vi "Grid Measurements - Topo & GridSpectr Simple.vi"(6 "Internal use":string, 7 "Grid param":T1 {"height (m)" format="%#_6p"; "width (m)" format="%#_6p"; "center Y (m)" format="%#_6p"; "center X (m)" format="%#_6p"}, 8 "Error in (no error)":errorcluster, 9 "Points Y/Index Y":i32, 10 "Points X/Index X":i32, 11 "Method":enum16{"init", "run", "end"}(ring)) -> (0 "Error out":errorcluster)   [LabVIEW 2014]
doc: "Example of a measurement VI to be used in the \"Experiments on a Grid\" tool as external VI.\n\nThis example measure the topography and spectroscopy data. The spectroscopy measurements are taken on a subgrid. The data are saved to a sxm and a binary file.\n\n- Nanonis Programming Interface -"
uses:
  Instance           1 53Saved   Grid Measurements Example - Topo & GridSpectr .vi
  <userlib>/Nanonis Prog Interface V5/Nanonis Prog Interface.lvlib
panel:
  out "Status":string
  out "Points taken":i32
  in  "Drift correction":i64
  in  "Y subgrid spacing":u16=4
  in  "X subgrid spacing":u16=4
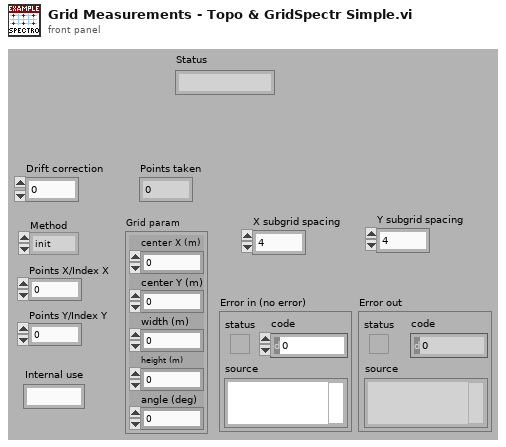
[diagram p1: front panel]
types:
  T1 = cluster{"center X (m)":sgl, "center Y (m)":sgl, "width (m)":sgl, "height (m)":sgl, "angle (deg)":sgl}
  T2 = cluster{"center X":sgl, "center Y":sgl, "angle":sgl, "width":sgl, "height":sgl, "# pixels":i32, "# lines":i32}
  T3 = cluster{"Name":string, "Calibration":sgl, "Offset":sgl, "Channel index":i32}[]
  T4 = cluster{"up/down":bool, "time/line":sgl, "start time":timestamp, "end time":timestamp}
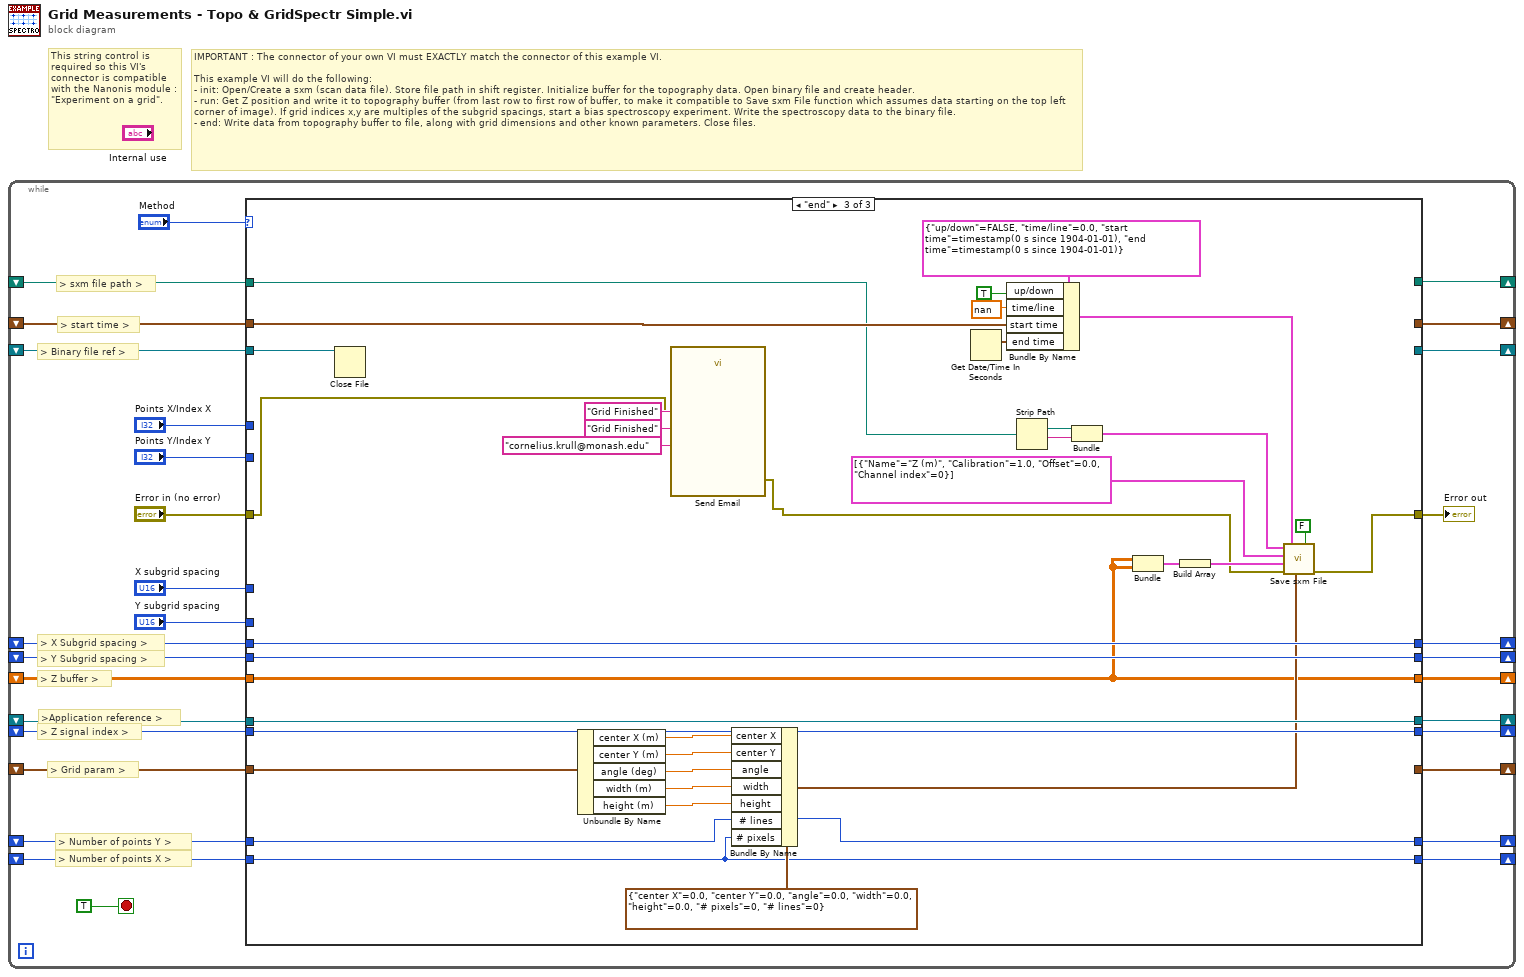
[diagram p0: block diagram]
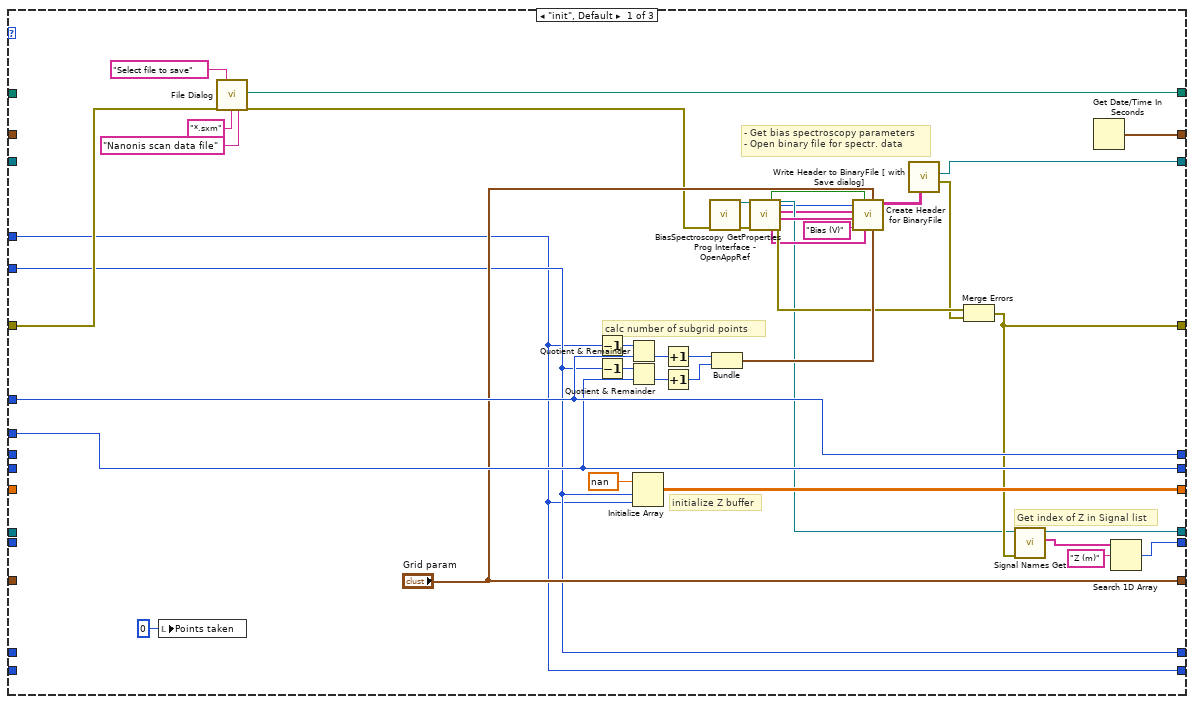
[diagram p2: hidden frame]
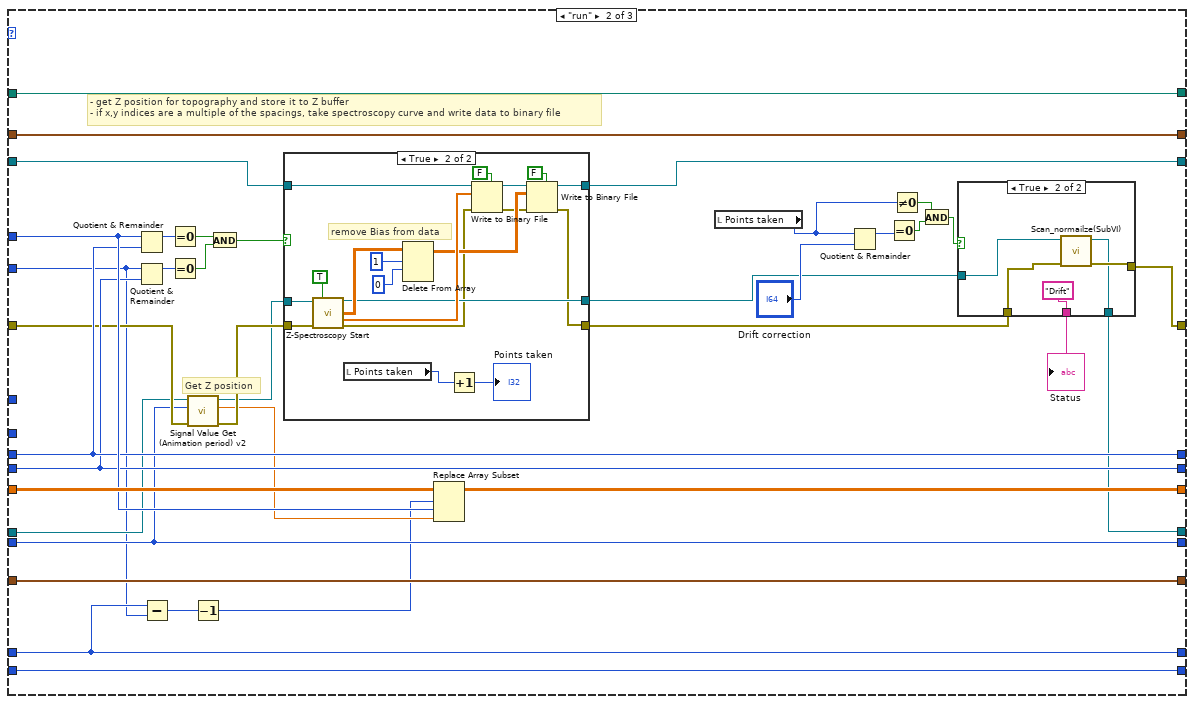
[diagram p3: hidden frame]
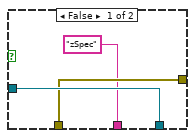
[diagram p4: hidden frame]
diagram:
  # "This string control is required so this VI's connector is compatible with the Nanonis module : \"Experiment on a grid\"."
  # "IMPORTANT : The connector of your own VI must EXACTLY match the connector of this example VI.\n\nThis example VI will do the following:\n- init: Open/Create a sxm (scan data file). Store file path in shift register. Initialize buffer for the topography data. Open binary file and create header.\n- run: Get Z position and write it to topography buffer (from last row to first row of buffer, to make it compatible to Save sxm File function which assumes data starting on the top left corner of image). If grid indices x,y are multiples of the subgrid spacings, start a bias spectroscopy experiment. Write the spectroscopy data to the binary file.\n- end: Write data from topography buffer to file, along with grid dimensions and other known parameters. Close files."
  n1 = while {
    shift-right: [w5] -> _
    shift-left: _ -> [w28]
    shift-right: [w23] -> _
    shift-left: _ -> [w22]
    shift-right: [w20] -> _
    shift-left: _ -> [w21]
    shift-right: [w19] -> _
    shift-left: _ -> [w18]
    shift-right: [w12] -> _
    shift-left: _ -> [w14]
    shift-right: [w13] -> _
    shift-left: _ -> [w15]
    shift-right: [w11] -> _
    shift-left: _ -> [w10]
    shift-right: [w9] -> _
    shift-left: _ -> [w8]
    shift-right: [w7] -> _
    shift-left: _ -> [w6]
    shift-right: [w4] -> _
    shift-left: _ -> [w3]
    shift-right: [w2] -> _
    shift-left: _ -> [w1]
    stop <- TRUE stop-if-true
    # "> Number of points X >"
    # "> Number of points Y >"
    # "> Grid param >"
    # "> start time >"
    # ">Application reference >"
    # "> Y Subgrid spacing >"
    # "> X Subgrid spacing >"
    # "> Z signal index >"
    # "> Binary file ref >"
    # "> Z buffer >"
    # "> sxm file path >"
    n2 = case shown="\"end\"" "Method" {
      tunnel: [w36 w107 _] -> w5
      tunnel: w28 -> [_ w107 w162]
      tunnel: "Error in (no error)" -> [w38 w94 w138]
      tunnel: [w48 w73 w154] -> w26
      tunnel: "Points X/Index X" -> [w32 w102 _]
      tunnel: "Points Y/Index Y" -> [w33 w84 _]
      tunnel: [w70 w105 w143] -> w23
      tunnel: w22 -> [_ w106 w143]
      tunnel: w21 -> [_ w104 w172]
      tunnel: [w61 w103 _] -> w20
      tunnel: [w59 w92 w173] -> w19
      tunnel: w18 -> [_ w92 w173]
      tunnel: "X subgrid spacing" -> [w58 _ _]
      tunnel: "Y subgrid spacing" -> [w57 _ _]
      tunnel: w15 -> [_ w96 w171]
      tunnel: w14 -> [_ w95 w170]
      tunnel: [w58 w96 w171] -> w13
      tunnel: [w57 w95 w170] -> w12
      tunnel: [w44 w72 w169] -> w11
      tunnel: w10 -> [_ w90 w169]
      tunnel: ["Grid param" w87 _] -> w9
      tunnel: w8 -> [_ w87 w153]
      tunnel: [w40 w88 _] -> w7
      tunnel: w6 -> [_ w88 w163]
      tunnel: [w33 w85 w144] -> w4
      tunnel: w3 -> [_ w85 w144]
      tunnel: [w32 w86 w145] -> w2
      tunnel: w1 -> [_ w86 w145]
      frame "init", Default {
        # "- Get bias spectroscopy parameters\n- Open binary file for spectr. data"
        # "initialize Z buffer"
        # "calc number of subgrid points"
        # "Get index of Z in Signal list"
        n3 = local write "Points taken"(0 ("Points taken")) -> ()
        n4 = call "File Dialog"("prompt"="Select file to save", "error in"=w38, "pattern (all files)"="*.sxm" ("pattern"), "pattern label"="Nanonis scan data file") -> ("selected path"=w36:path, "error out"=w37:errorcluster)  [unwired: 8 in, 2 out]
        n5 = Decrement(x=w32) -> (x-1=w56:i32)
        n6 = Decrement(x=w33) -> (x-1=w55:i32)
        n7 = Quotient & Remainder(x=w56, y=w58) -> (floor(x/y)=w54:i32)  [unwired: 1 out]
        n8 = Quotient & Remainder(x=w55, y=w57) -> (floor(x/y)=w53:i32)  [unwired: 1 out]
        n9 = Initialize Array(sgl nan ("element"), w33, w32) -> (w70:sgl[][])
        n10 = Increment(x=w54) -> (x+1=w52:i32)
        n11 = Increment(x=w53) -> (x+1=w51:i32)
        n12 = call <userlib>:"Prog Interface - OpenAppRef.vi"("Error in (no error)"=w37) -> ("Error out"=w49:errorcluster, "Application reference"=w47:refnum<vi>)  [unwired: 5 in]
        n13 = Bundle(w52, w51) -> (w65:cluster{i32, i32})  [unwired: 1 in]
        n14 = call <userlib>:"BiasSpectroscopy GetProperties.vi"("Application ref in"=w47, "Error in (no error)"=w49) -> ("Backward sweep"=w66:bool, "Application ref out"=w46:refnum<vi>, "Number of points"=w43:i32, "Channels"=w42:string[], "Parameters"=w64:string[], "Fixed parameters"=w50:string[], "Error out"=w63:errorcluster)  [unwired: 5 in, 2 out]
        n15 = call <userlib>:"Create Header for BinaryFile.vi"("Grid points"=w65, "Grid param"="Grid param", "Fixed parameters"=w50, "Backward sweep"=w66, "Sweep signal"="Bias (V)" ("Sweep Signal"), "Parameters"=w64, "Channels"=w42, "Points per sweep"=w43) -> ("Header (fixed attributes)"=w68:string[][])  [unwired: 3 in]
        n16 = call <userlib>:"Write Header to BinaryFile [ with Save dialog].vi"("Fixed Attributes"=w68) -> ("Error out"=w62:errorcluster, "File ref"=w61:refnum<file>)  [unwired: 7 in, 2 out]
        n17 = Merge Errors(w63, w62) -> (w48:errorcluster)
        n18 = call <userlib>:"Signal Names Get.vi"("error in (no error)"=w48, "Application ref in"=w46) -> ("Signals Names"=w45:string[], "Application ref out"=w44:refnum<vi>)  [unwired: 5 in, 1 out]
        n19 = Get Date/Time In Seconds() -> (seconds since 1Jan1904=w40:timestamp)
        n20 = Search 1D Array(1D array=w45, element="Z (m)") -> (index of element=w59:i32)  [unwired: 1 in]
      }
      frame "run" {
        # "Get Z position"
        # "- get Z position for topography and store it to Z buffer\n- if x,y indices are a multiple of the spacings, take spectroscopy curve and write data to binary file"
        n21 = Quotient & Remainder(x=w102, y=w96) -> (x-y*floor(x/y)=w101:i32)  [unwired: 1 out]
        n22 = Quotient & Remainder(x=w84, y=w95) -> (x-y*floor(x/y)=w100:i32)  [unwired: 1 out]
        n23 = Subtract(x=w85, y=w84) -> (x-y=w83:i32)
        n24 = Equal To 0?(x=w101) -> (x = 0?=w99:bool)
        n25 = Equal To 0?(x=w100) -> (x = 0?=w98:bool)
        n26 = call <userlib>:"Signal Value Get (Animation period) v2.vi"("error in (no error)"=w94, "Signal index (0-79)"=w92, "Application ref in"=w90) -> ("error out"=w93:errorcluster, "Signal value"=w91:sgl, "Application ref out"=w89:refnum<vi>)  [unwired: 5 in]
        n27 = Decrement(x=w83) -> (x-1=w82:i32)
        n28 = And(x=w99, y=w98) -> (x .and. y?=w97:bool)
        n29 = case shown="True" w97 {
          tunnel: [w117 w121] -> w74
          tunnel: w104 -> [w118 w137]
          tunnel: [w118 w135] -> w103
          tunnel: w93 -> [w117 w134]
          tunnel: w89 -> [w116 w126]
          tunnel: [w116 w125] -> w75
          frame False {
            # "Point indices aren't multiple of subgrid spacing\n=> no spectroscopy at this point"
          }
          frame True {
            # "remove Bias from data"
            n30 = call <userlib>:"Z-Spectroscopy Start.vi"("Application ref in"=w126, "Get data (F=False)"=TRUE ("Get Data (F)"), "error in (no error)"=w134) -> ("Application ref out"=w125:refnum<vi>, "Data"=w133:sgl[][], "Parameters"=w132:sgl[], "error out"=w123:errorcluster)  [unwired: 8 in, 1 out]
            n31 = local read "Points taken"() -> (w120:i32)
            n32 = Delete From Array(array=w133, length=1, index (row)=0 ("index")) -> (array with subset deleted=w131:sgl[][])  [unwired: 1 in, 1 out]
            n33 = Increment(x=w120) -> (x+1=→"Points taken":i32)
            n34 = Write to Binary File(file (use dialog)=w137, data=w132, error in=w123, 5:FALSE ("prepend array or string size? (T)")) -> (refnum out=w136:refnum<file>, error out=w122:errorcluster)  [unwired: 2 in, 1 out]
            n35 = Write to Binary File(file (use dialog)=w136, data=w131, error in=w122, 5:FALSE ("prepend array or string size? (T)")) -> (refnum out=w135:refnum<file>, error out=w121:errorcluster)  [unwired: 2 in, 1 out]
          }
        }
        n36 = Replace Array Subset(array=w106, new element=w91, index (row)=w82, index (col)=w102) -> (w105:sgl[][])
        n37 = local read "Points taken"() -> (w79:i32)
        n38 = Quotient & Remainder(x=w79, y="Drift correction") -> (x-y*floor(x/y)=w80:i64)  [unwired: 1 out]
        n39 = Equal To 0?(x=w80) -> (x = 0?=w77:bool)
        n40 = Not Equal To 0?(x=w79) -> (x != 0?=w78:bool)
        n41 = And(x=w78, y=w77) -> (x .and. y?=w76:bool)
        n42 = case shown="True" w76 {
          tunnel: w75 -> [w110 w113]
          tunnel: w74 -> [w109 w112]
          tunnel: [w109 w115] -> w73
          tunnel: [w110 w114] -> w72
          tunnel: ["zSpec" ("Status") "Drift" ("Status")] -> w71
          frame False {
          }
          frame True {
            n43 = call "Scan_normailze(SubVI).vi"("error in (no error)"=w112, "Application in"=w113) -> ("error out"=w115:errorcluster, "Application out"=w114:refnum<vi>)  [unwired: 7 in, 1 out]
          }
        }
        "Status" <- w71
      }
      frame "end" {
        n44 = Close File(refnum=w172) -> ()  [unwired: 1 in, 2 out]
        n45 = Unbundle By Name(w153) -> ("center X (m)"=w151:sgl, "center Y (m)"=w150:sgl, "angle (deg)"=w149:sgl, "width (m)"=w148:sgl, "height (m)"=w147:sgl)
        n46 = call "Send Email"("error in"=w138, "Message"="Grid Finished", "Subject"="Grid Finished", "Recipients"="cornelius.krull@monash.edu") -> ("error out"=w139:errorcluster)  [unwired: 7 in]
        n47 = Bundle By Name(cluster=T2 {"center X"=0.0, "center Y"=0.0, "angle"=0.0, "width"=0.0, "height"=0.0, "# pixels"=0, "# lines"=0} ("Scanfield"), "center X"=w151, "center Y"=w150, "angle"=w149, "width"=w148, "height"=w147, "# lines"=w144, "# pixels"=w145) -> (w146:T2)
        n48 = Get Date/Time In Seconds() -> (seconds since 1Jan1904=w160:timestamp)
        n49 = Bundle By Name(cluster=T4 {"up/down"=FALSE, "time/line"=0.0, "start time"=timestamp(0 s since 1904-01-01), "end time"=timestamp(0 s since 1904-01-01)} ("Scan param"), "up/down"=TRUE, "time/line"=sgl nan ("input 7"), "start time"=w163, "end time"=w160) -> (w161:T4)
        n50 = Strip Path(path=w162) -> (stripped path=w157:path, name=w156:string)
        n51 = Bundle("stripped path"=w157, "name"=w156) -> (w155:cluster{"stripped path":path, "name":string})  [unwired: 1 in]
        n52 = Bundle(w143, w143) -> (w168:cluster{sgl[][], sgl[][]})  [unwired: 1 in]
        n53 = Build Array(w168) -> (w167:cluster{sgl[][], sgl[][]}[])
        n54 = call <userlib>:"Save sxm File.vi"("Auto file naming? (T)"=FALSE, "Scanfield"=w146, "Scan param"=w161, "error in (no error)"=w139, "Channels data"=w167, "Channels config"=T3 [{"Name"="Z (m)", "Calibration"=1.0, "Offset"=0.0, "Channel index"=0}], "Filename control"=w155) -> ("error out"=w154:errorcluster)  [unwired: 2 in, 2 out]
      }
    }
    "Error out" <- w26
  }
